vi "[GV]_LIDAR Port NUM.vi"() -> ()   [LabVIEW 2016]
panel:
  in  "Lidar port number":u16=2111
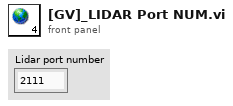
[diagram p1: front panel]
diagram:
